vi "RP proccess I-V.vi"() -> ()   [LabVIEW 2024]
uses:
  <vilib>/Analysis/NI_AALPro.lvlib
  Utilities/Fit/Smooth Background WFRM DBL.vi
  Waform generation/I-V parameters.ctl
panel:
  in  "HP F":dbl=nan format="%#_6pHz"
  in  "LP  Frequency":dbl=nan format="%#_6pHz"
  in  "I-V parameters":T1={"Start magnitude"=0.01, "Magnitude increment"=0.001, "End magnitude"=8.0, "Ramp length"=32, "Top  length"=224, "Threshold "=1e-05, "Processing delay"=132, "Output gain "=224.0, "Interpolation"=64, "Stop after"=0, "Detector window"=480} {"Detector window" format="%dpts"; "Stop after" format="%d sweep(s)"; "Output gain" format="%#_6pA/V"; "Processing delay" format="%dpts"; "Threshold" format="%#_6pV"; "Top  length" format="%dpts"; "Ramp length" format="%dpts"; "End magnitude" format="%#_6pA"; "Magnitude increment" format="%#_6pA"; "Start magnitude" format="%#_6pA"}
  in  "Signal ch":string="CH0"
  in  "Current ch":string="CH1"
  in  "Field tiime shift":dbl=0.0096 format="%#_6p"
  in  "Save output":bool
  in  "Integrate Bdot":bool
  out "XY Graph":cluster{dbl[], "Y":dbl[]}[](graph)
  out "Error Out":errorcluster
  in  "Bdot calibration":dbl=2506.0
  in  "offset length":i32=990000
  out "Waveform Graph":waveform(dbl)[](graph)
  in  "B channel":string="Field_fixed"
  in  "Avg V channel":string="Avg Volts"
  in  "Field":path
  in  "Signal file":path
  # "Waveform parameters"
  # "Detector parameters"
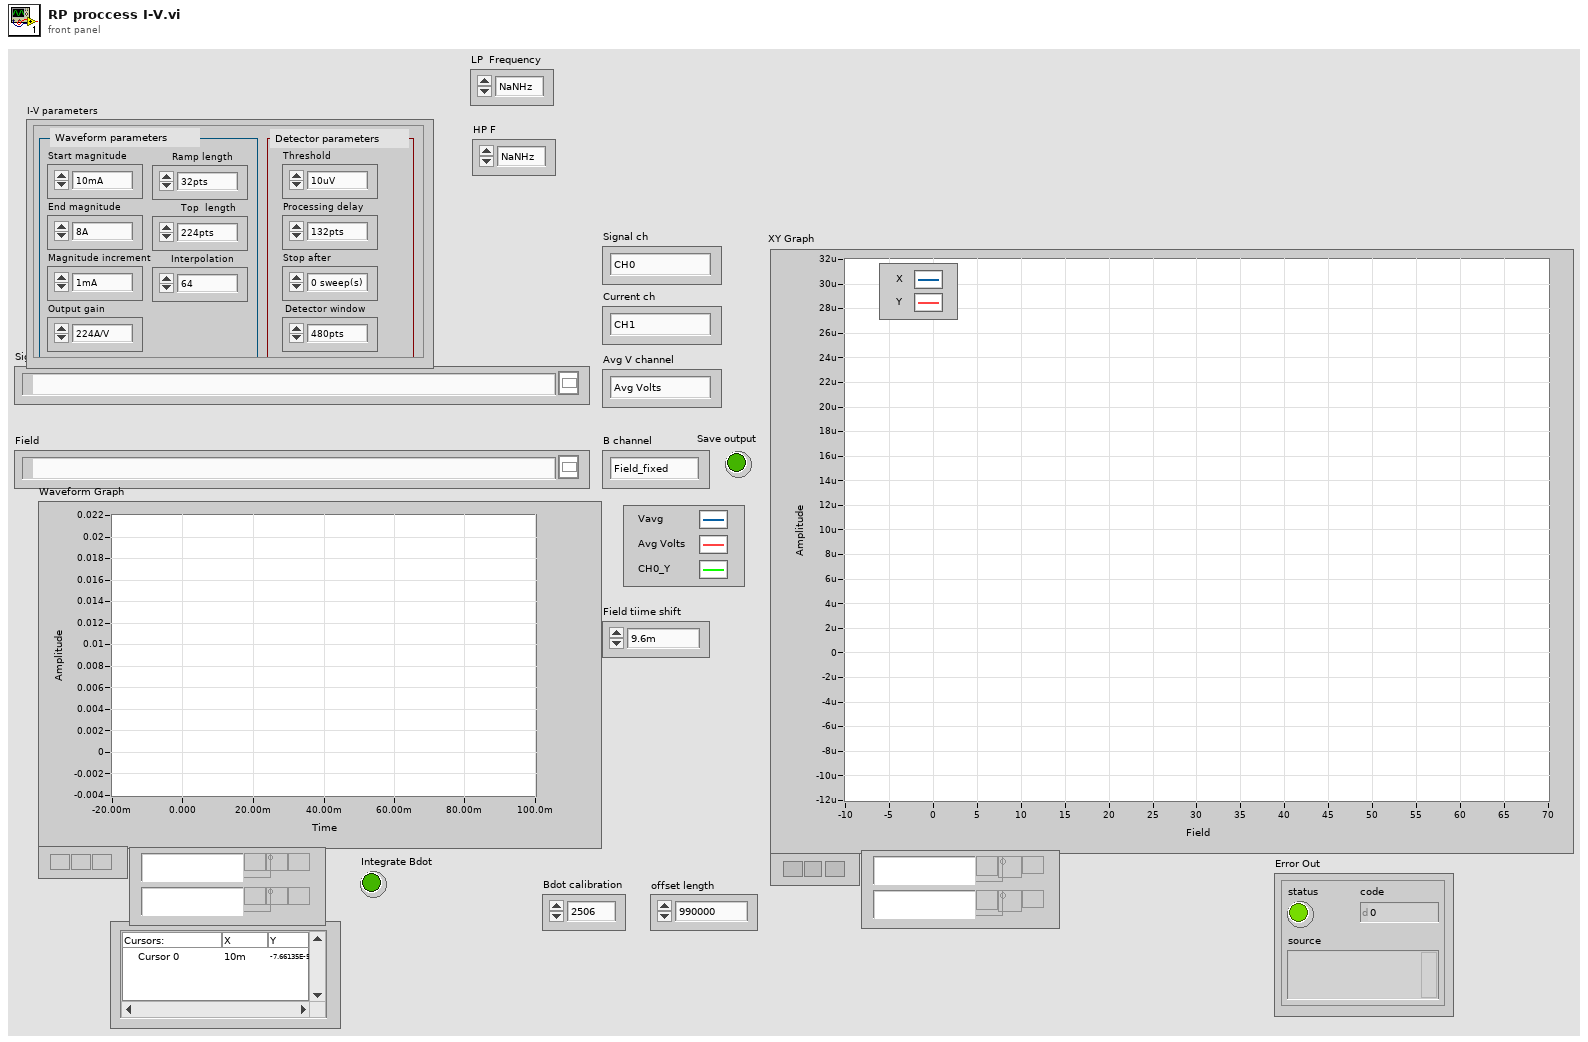
[diagram p1: front panel]
types:
  T1 = typedef "I-V parameters.ctl" = cluster{"Start magnitude":dbl, "Magnitude increment":dbl, "End magnitude":dbl, "Ramp length":i32, "Top  length":i32, "Threshold ":dbl, "Processing delay":u16, "Output gain ":dbl, "Interpolation":i32, "Stop after":u16, "Detector window":i32}
  T2 = enum16{"open", "open or create", "create or replace", "create", "open (read-only)"}
  T3 = cluster{"Waveform":waveform(dbl), "Waveform":waveform(dbl)}
  T4 = cluster{"Waveform":waveform(dbl), "Waveform":waveform(dbl)}[]
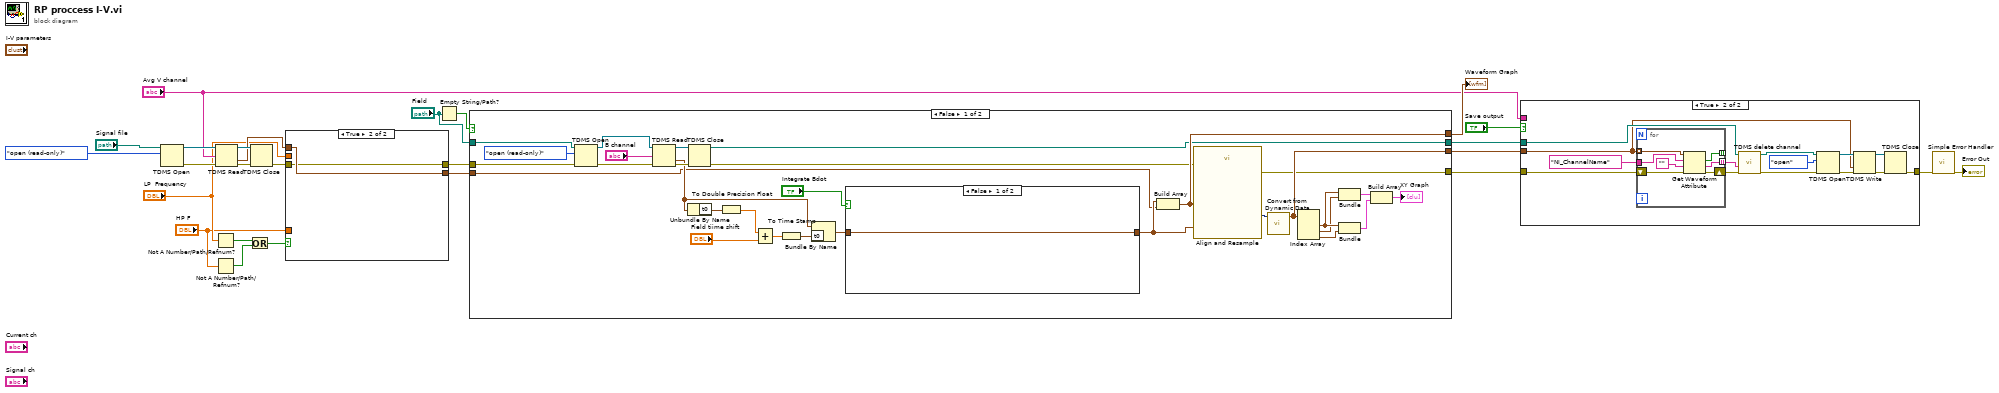
[diagram p0: block diagram]
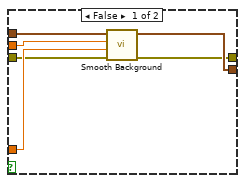
[diagram p2: hidden frame]
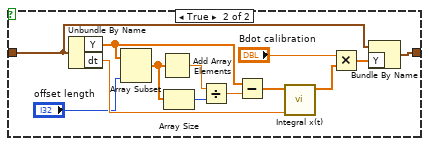
[diagram p3: hidden frame]
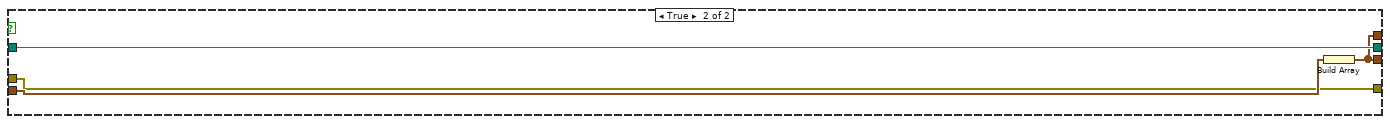
[diagram p4: hidden frame]
diagram:
  n1 = TDMS Open(10:T2."open (read-only)" ("operation (0:open)"), 11:"Signal file") -> (0:w14:errorcluster, 3:w15:refnum<k34>)  [unwired: 5 in]
  n2 = Not A Number/Path/Refnum?(number/path/refnum="LP  Frequency") -> (NaN/Path/Refnum?=w3:bool)
  n3 = Not A Number/Path/Refnum?(number/path/refnum="HP F") -> (NaN/Path/Refnum?=w2:bool)
  n4 = TDMS Read(0:w15, 7:"Avg V channel", 11:w14) -> (4:w17:refnum<k34>, 10:w9:waveform(dbl), 15:w16:errorcluster)  [unwired: 5 in, 3 out]
  n5 = Or(x=w3, y=w2) -> (x .or. y?=w1:bool)
  n6 = TDMS Close(8:w16, 11:w17) -> (0:w7:errorcluster)  [unwired: 1 out]
  n7 = case shown="True" w1 {
    tunnel: w9 -> [w31 w33]
    tunnel: [w30 w33] -> w8
    tunnel: "LP  Frequency" -> [w29 _]
    tunnel: "HP F" -> [w28 _]
    tunnel: w7 -> [w27 w32]
    tunnel: [w26 w32] -> w6
    frame False {
      n8 = call-poly "Smooth Background.vi"("Error In"=w27, "HP F"=w28, "LP  F"=w29, "Data"=w31) -> ("Error Out"=w26:errorcluster, "Data out"=w30:waveform(dbl))  [unwired: 6 in]
    }
    frame True {
    }
  }
  n9 = Empty String/Path?(string/path="Field") -> (empty?=w19:bool)
  n10 = case shown="False" w19 {
    tunnel: w8 -> [w34 w81]
    tunnel: [w50 w78] -> w25
    tunnel: [w49 w80] -> w23
    tunnel: [w46 w78] -> w21
    tunnel: "Field" -> [w45 w80]
    tunnel: w6 -> [w42 w79]
    tunnel: [w43 w79] -> w18
    frame False {
      n11 = TDMS Open(8:w42, 10:T2."open (read-only)" ("operation (0:open)"), 11:w45) -> (0:w62:errorcluster, 3:w61:refnum<k34>)  [unwired: 4 in]
      n12 = TDMS Read(0:w61, 7:"B channel", 11:w62) -> (4:w58:refnum<k34>, 10:w36:waveform(dbl), 15:w59:errorcluster)  [unwired: 5 in, 3 out]
      n13 = Unbundle By Name(w36) -> ("t0"=w41:timestamp)
      n14 = TDMS Close(8:w59, 11:w58) -> (0:w44:errorcluster, 3:w49:path)
      n15 = To Double Precision Float(number=w41) -> (double precision float=w40:dbl)
      n16 = Add(x=w40, y="Field tiime shift") -> (x+y=w38:dbl)
      n17 = To Time Stamp(1:w38) -> (0:w37:timestamp)
      n18 = Bundle By Name(cluster=w36, "t0"=w37) -> (w35:waveform(dbl))
      n19 = case shown="False" "Integrate Bdot" {
        tunnel: w35 -> [w64 w67]
        tunnel: [w64 w65] -> w56
        frame False {
        }
        frame True {
          n20 = Unbundle By Name(w67) -> ("Y"=w70:dbl[], "dt"=w77:dbl)
          n21 = Array Subset(array=w70, length="offset length") -> (w74:dbl[])  [unwired: 1 in]
          n22 = Add Array Elements(numeric array=w74) -> (sum=w73:dbl)
          n23 = Array Size(array=w74) -> (size(s)=w72:i32)
          n24 = Divide(x=w73, y=w72) -> (x/y=w69:dbl)
          n25 = Subtract(x=w70, y=w69) -> (x-y=w71:dbl[])
          n26 = call <vilib>:"Integral x(t).vi"("dt"=w77, "X"=w71) -> ("Integral X"=w76:dbl[])  [unwired: 8 in, 1 out]
          n27 = Multiply(x="Bdot calibration", y=w76) -> (x*y=w66:dbl[])
          n28 = Bundle By Name(cluster=w67, "Y"=w66) -> (w65:waveform(dbl))
        }
      }
      n29 = Build Array(w56, w34) -> (w50:waveform(dbl)[])
      n30 = call "Align and Resample"("Reference Signal"=w56, "error in (no error)"=w44, "Signals"=w50) -> ("error out"=w43:errorcluster, "Resampled Signals"=w55:dynamicdata)  [unwired: 6 in, 1 out]
      n31 = call "Convert from Dynamic Data"("Dynamic Data Type"=w55) -> ("Array of Waveform"=w46:waveform(dbl)[])  [unwired: 3 in]
      n32 = Index Array(array=w46) -> (element #1=w54:waveform(dbl), element #2=w48:waveform(dbl), element #3=w47:waveform(dbl))  [unwired: 3 in]
      n33 = Bundle("Waveform"=w54, "Waveform"=w48) -> (w53:T3)  [unwired: 1 in]
      n34 = Bundle("Waveform"=w54, "Waveform"=w47) -> (w52:T3)  [unwired: 1 in]
      n35 = Build Array(w53, w52) -> (→"XY Graph":T4)
    }
    frame True {
      n36 = Build Array(w81) -> (w78:waveform(dbl)[])
    }
  }
  "Waveform Graph" <- w25
  n37 = case shown="True" "Save output" {
    tunnel: w23 -> [_ w92]
    tunnel: w18 -> [w82 w86]
    tunnel: [w82 w94] -> w22
    tunnel: "Avg V channel" -> [_ _]
    tunnel: w21 -> [_ w83]
    frame False {
    }
    frame True {
      n38 = for {
        tunnel: w83 -> [w103] mode=indexing
        tunnel: "NI_ChannelName" ("name") -> [w102]
        tunnel: [w101] -> _ mode=indexing
        tunnel: [w97] -> w84 mode=indexing
        shift-right: [w99] -> w85
        shift-left: w86 -> [w100]
        n39 = Get Waveform Attribute(4:w100, 5:"", 6:w102, 7:w103) -> (0:w99:errorcluster, 1:w97:string, 2:w101:bool)  [unwired: 1 out]
      }
      n40 = call "TDMS delete channel.vi"("error in (no error)"=w85, "Channels"=w84, "file path"=w92) -> ("error out"=w91:errorcluster, "file path out"=w90:path)  [unwired: 6 in, 1 out]
      n41 = TDMS Open(8:w91, 10:T2."open" ("operation (0:open)"), 11:w90) -> (0:w88:errorcluster, 3:w89:refnum<k34>)  [unwired: 4 in]
      n42 = TDMS Write(0:w89, 9:w83, 11:w88) -> (4:w96:refnum<k34>, 15:w95:errorcluster)  [unwired: 3 in, 2 out]
      n43 = TDMS Close(8:w95, 11:w96) -> (0:w94:errorcluster)  [unwired: 1 out]
    }
  }
  n44 = call <vilib>:"Simple Error Handler.vi"("error in (no error)"=w22) -> ("error out"=→"Error Out":errorcluster)  [unwired: 4 in, 4 out]
